vi "myRIO_BRig_RT_dataCurrent_iBlock.vi"() -> (2 "output_iBlock":i32)   [LabVIEW 2014]
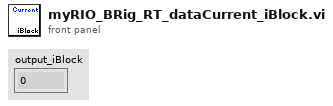
[diagram p1: front panel]
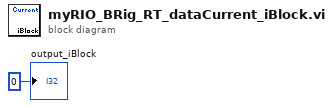
[diagram p0: block diagram]
diagram:
  "output_iBlock" <- 0 ("output_iBlock")
